vi "Get Filename Offset.vi"(8 "error in (no error)":errorcluster, 11 "Log File Specification in":refnum<class "Log File Specification.lvclass">) -> (0 "error out":errorcluster, 2 "Filename Offset":i32, 3 "Log File Specification out":refnum<class "Log File Specification.lvclass">)   [LabVIEW 2015, in "Log File Specification.lvclass"]
doc: "Gets the filename offset, which is the first number appended to a filename in case of a conflict if the Create Unique File Path option is set. Setting this number can help reduce the number of tries it takes to find a unique file path."
uses:
  Log File Specification.lvclass
  Log File Specification.lvclass/Log File Specification.ctl
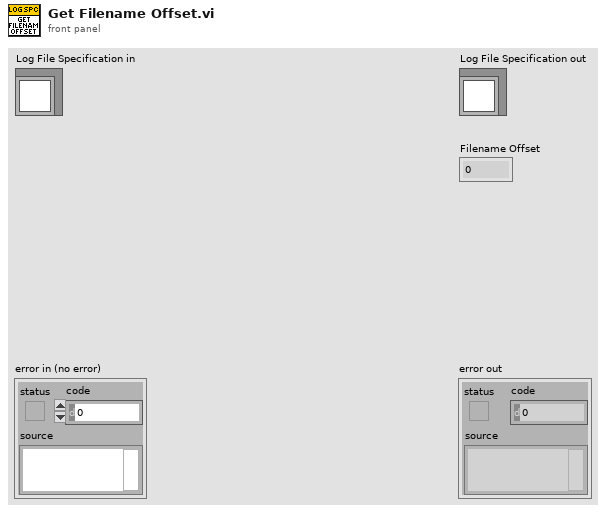
[diagram p1: front panel]
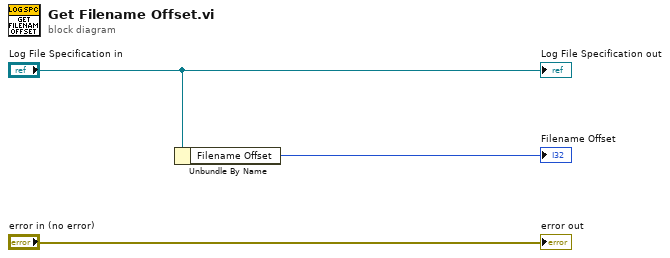
[diagram p0: block diagram]
diagram:
  n1 = Unbundle By Name("Log File Specification in") -> ("Filename Offset"=→"Filename Offset":i32)
  "error out" <- "error in (no error)"
  "Log File Specification out" <- "Log File Specification in"
